vi "Grab.vi"() -> ()   [LabVIEW 2017]
doc: "The Grab VI acquires images continuously and displays the images in an image control using high-level acquisition VIs. A grab is appropriate for high-speed applications in which you need to process only one image at a time."
uses:
  <vilib>/vision/driver/NI_Vision_Acquisition_Software.lvlib
panel:
  in  "UI电源线正面标签1参数 2":T2={"Rectangle"={"Left"=1066, "Top"=596, "Right"=370, "Bottom"=2690, "Rotation"=45.0}, "Angle (degrees) (Geometry 1)"=90.0, "中心位置"={"Cent X"=273.0, "Cent Y"=255.0, "半径"=300.0}, "long"=150.0, "abgek"=-90.0, "Color"=16711680, "left threshold"=0.0, "Rectangle right"={"Left"=1066, "Top"=1096, "Right"=570, "Bottom"=2690, "Rotation"=45.0}, "long right"=150.0, "abgek right"=90.0, "Color 2"=16711680, "right threshold"=0.0, "left"=0.0, "right"=0.0} {"Rectangle right"."Rotation" format="%.2f"; "Rectangle right"."Left" scale=0.0..1024.0; "Rectangle right"."Right" scale=0.0..1024.0; "Rectangle"."Rotation" format="%.2f"; "Rectangle"."Left" scale=0.0..1024.0; "Rectangle"."Right" scale=0.0..1024.0}
  out "输出簇":T3={"Clamp Points (Max Clamp 1)"={"Pixels "={"Start"={"X"=804.5, "Y"=852.5074462890625}, "End"={"X"=804.5, "Y"=932.54296875}}, "Real World"={"Start"={"X"=804.5, "Y"=852.5074462890625}, "End"={"X"=804.5, "Y"=932.54296875}}}, "Clamp Points (Max Clamp 2)"={"Pixels "={"Start"={"X"=1018.1555786132812, "Y"=879.031982421875}, "End"={"X"=1027.8096923828125, "Y"=907.3988647460938}}, "Real World"={"Start"={"X"=1018.1555786132812, "Y"=879.031982421875}, "End"={"X"=1027.8096923828125, "Y"=907.3988647460938}}}}
  in  "布尔":bool
  in  "等待时间（毫秒）":u32
  out "error out":errorcluster={"status"=TRUE, "code"=-1074396120, "source"="IMAQ WriteJPEGFile\n  "}
  in  "error in (no error)":errorcluster
  out "连接的字符串":string="\\20181121\\CCD2\\Image\\11_24_49.jpeg"
  in  "Camera Name":refnum<k21> caption="IMAQdx Session"
  out "Buffer Number":u32
  out "Image":T4(plugin-control)
  out "Frame Rate":dbl(knob) scale=0.0..100.0
  in  "Stop":bool
  # "Overview: Demonstrates how to acquire images continuously using a Grab acquisition.\nRequirements: Vision Acquisition Software\nInstructions: \n1. Select the Camera Name.\n2. Run the VI"
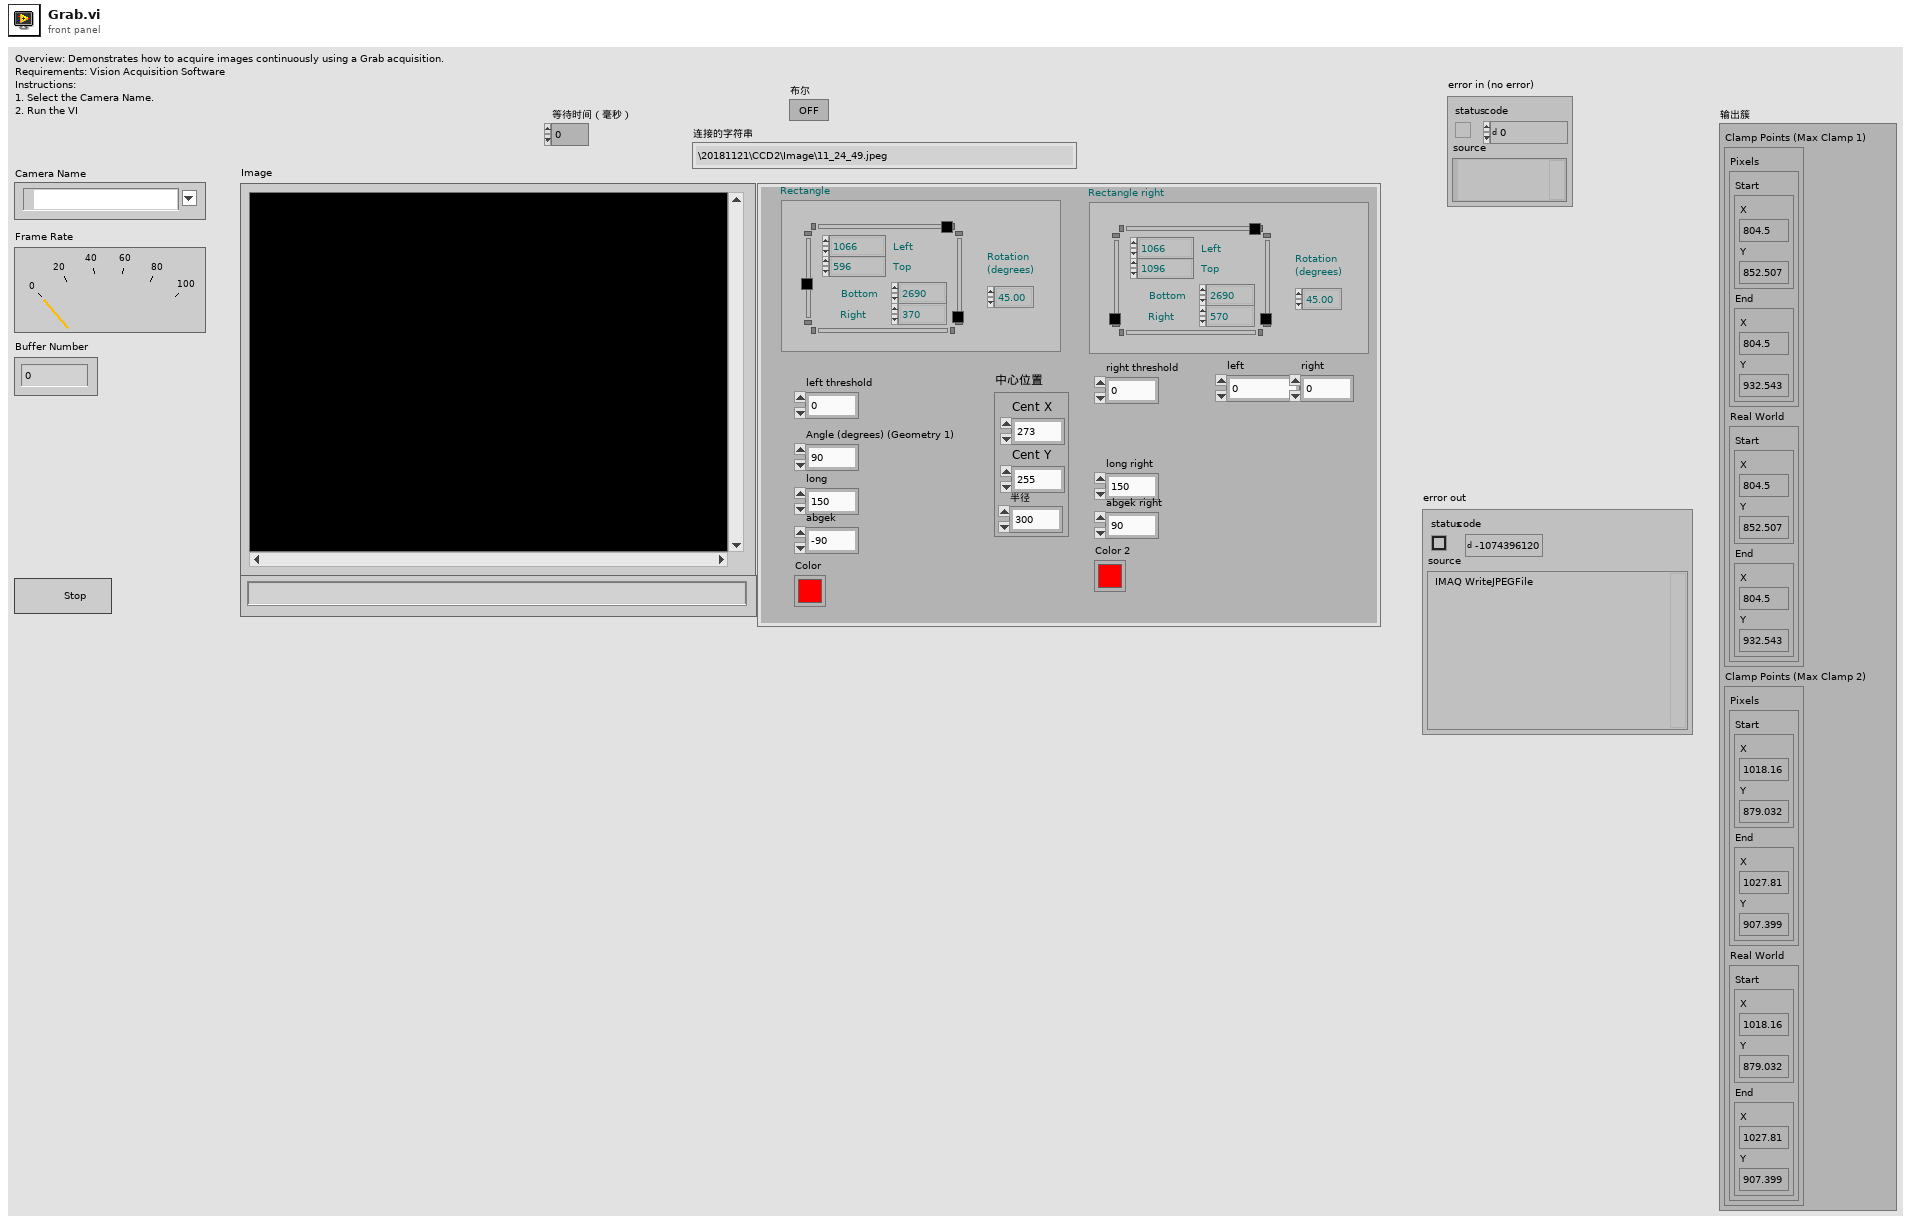
[diagram p1: front panel]
types:
  T1 = typedef "IMAQ Rectangle" = cluster{"Left":i32, "Top":i32, "Right":i32, "Bottom":i32, "Rotation":dbl}
  T2 = cluster{"Rectangle":T1, "Angle (degrees) (Geometry 1)":sgl, "中心位置":cluster{"Cent X":dbl, "Cent Y":dbl, "半径":dbl}, "long":sgl, "abgek":dbl, "Color":u32, "left threshold":dbl, "Rectangle right":T1, "long right":sgl, "abgek right":dbl, "Color 2":u32, "right threshold":dbl, "left":dbl, "right":dbl}
  T3 = cluster{"Clamp Points (Max Clamp 1)":cluster{"Pixels ":cluster{"Start":cluster{"X":dbl, "Y":dbl}, "End":cluster{"X":dbl, "Y":dbl}}, "Real World":cluster{"Start":cluster{"X":dbl, "Y":dbl}, "End":cluster{"X":dbl, "Y":dbl}}}, "Clamp Points (Max Clamp 2)":cluster{"Pixels ":cluster{"Start":cluster{"X":dbl, "Y":dbl}, "End":cluster{"X":dbl, "Y":dbl}}, "Real World":cluster{"Start":cluster{"X":dbl, "Y":dbl}, "End":cluster{"X":dbl, "Y":dbl}}}}
  T4 = typedef "IMAQ Image.ctl" = refnum<image>
  T5 = typedef "IMAQdx.ctl" = refnum<k21>
  T6 = cluster{"Pixels ":cluster{"Start":cluster{"X":dbl, "Y":dbl}, "End":cluster{"X":dbl, "Y":dbl}}, "Real World":cluster{"Start":cluster{"X":dbl, "Y":dbl}, "End":cluster{"X":dbl, "Y":dbl}}}
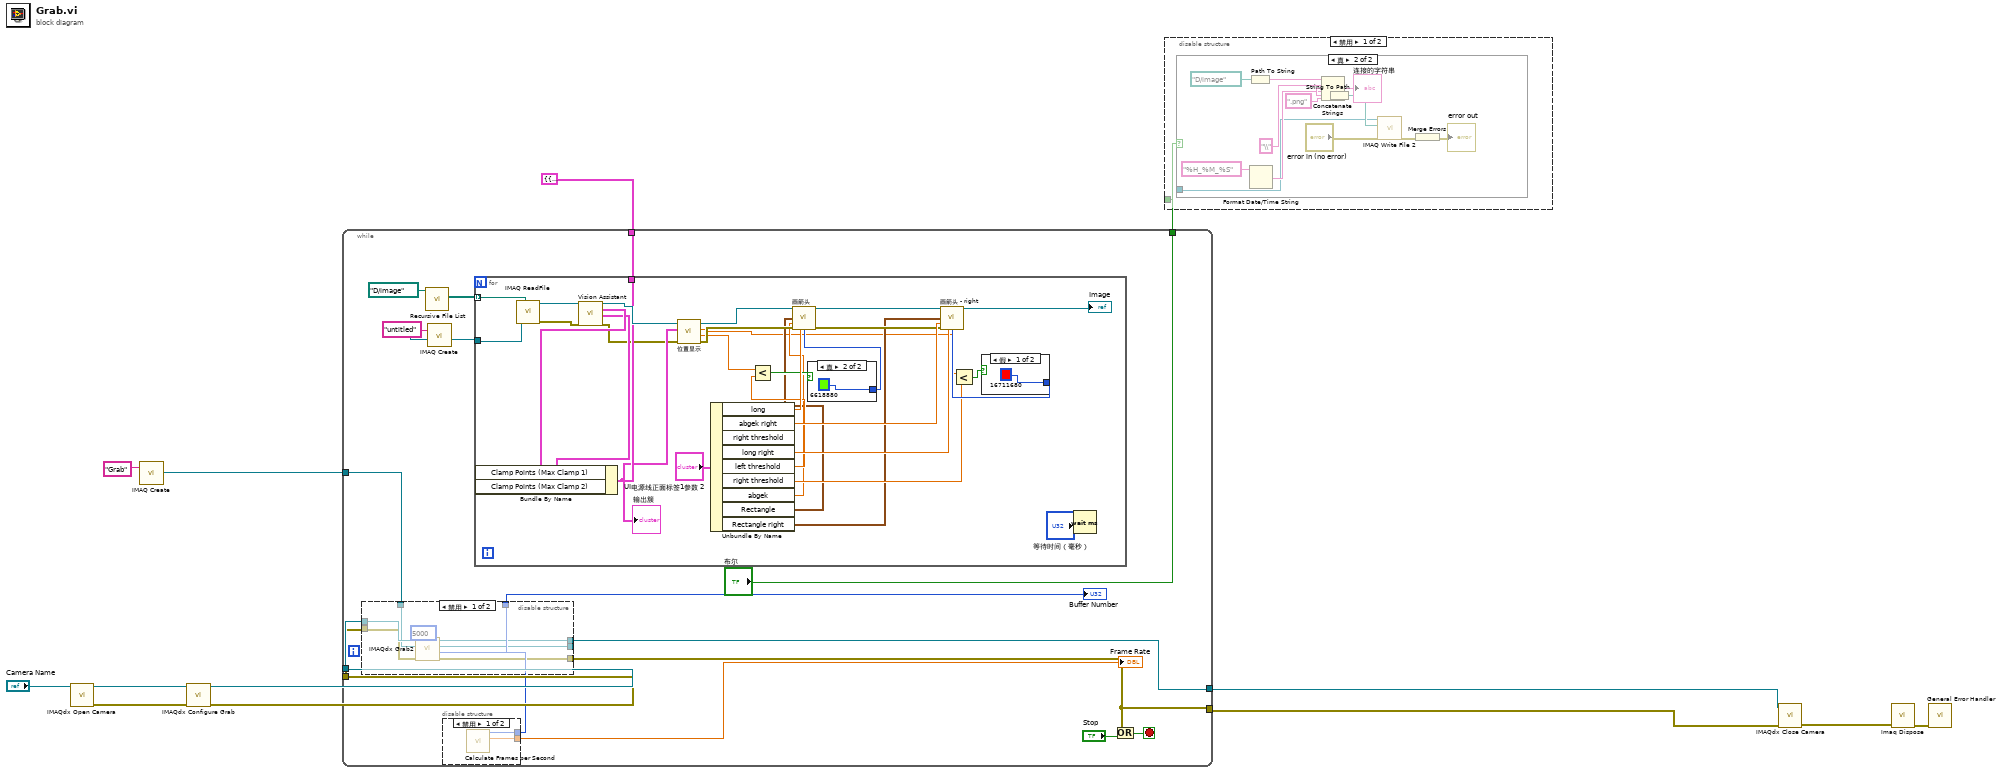
[diagram p0: block diagram]
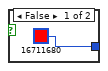
[diagram p4: hidden frame]
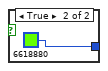
[diagram p5: hidden frame]
diagram:
  n1 = call <vilib>:"IMAQdx Open Camera.vi"("Session In"="Camera Name") -> ("error out"=w9:errorcluster, "Session Out"=w8:T5)  [unwired: 2 in, 7 out]
  n2 = call "IMAQ Create"("Image Name"="Grab") -> ("New Image"=w13:T4)  [unwired: 3 in, 2 out]
  n3 = call <vilib>:"IMAQdx Configure Grab.vi"("error in"=w9, "Session In"=w8) -> ("error out"=w11:errorcluster, "Session Out"=w12:T5)  [unwired: 8 out]
  n4 = while {
    tunnel: [w20] -> w3
    tunnel: w11 -> [w25]
    tunnel: w12 -> [w26]
    tunnel: [w21] -> w10
    tunnel: w13 -> [w24]
    tunnel: T3 {"Clamp Points (Max Clamp 1)"={"Pixels "={"Start"={"X"=0.0, "Y"=0.0}, "End"={"X"=0.0, "Y"=0.0}}, "Real World"={"Start"={"X"=0.0, "Y"=0.0}, "End"={"X"=0.0, "Y"=0.0}}}, "Clamp Points (Max Clamp 2)"={"Pixels "={"Start"={"X"=0.0, "Y"=0.0}, "End"={"X"=0.0, "Y"=0.0}}, "Real World"={"Start"={"X"=0.0, "Y"=0.0}, "End"={"X"=0.0, "Y"=0.0}}}} ("簇") -> [w15]
    tunnel: ["布尔"] -> w1
    stop <- w28 stop-if-true
    n5 = disable-structure shown="禁用" {
      disable-tunnel: w26 -> [w71 _]
      disable-tunnel: w25 -> [w70 _]
      disable-tunnel: w24 -> [w69 _]
      disable-tunnel: [w68 _] -> w22
      disable-tunnel: [w67 _] -> w21
      disable-tunnel: [w66 _] -> w20
      disable-tunnel: [w64 _] -> _
      frame Disabled {
        n6 = call <vilib>:"IMAQdx Grab2.vi"("Timeout (ms)"=5000, "error in"=w70, "Image In"=w69, "Session In"=w71) -> ("error out"=w67:errorcluster, "Buffer Number Out"=w68:u32, "Image Out"=w64:T4, "Session Out"=w66:T5)  [unwired: 4 in]
      }
      frame Enabled {
      }
    }
    "Buffer Number" <- w22
    n7 = call <vilib>:"Recursive File List.vi"("Folder Path"=path "D:/image") -> ("All Files in Dir"=w18:path[])  [unwired: 6 in, 4 out]
    n8 = call "IMAQ Create"("Image Name"="untitled") -> ("New Image"=w16:T4)  [unwired: 4 in, 1 out]
    n9 = disable-structure shown="禁用" {
      disable-tunnel: [w73 _] -> w23
      disable-tunnel: w22 -> [w72 _]
      frame Disabled {
        n10 = call <vilib>:"Calculate Frames per Second.vi"("Buffer Number"=w72) -> ("Processed Frames/s"=w73:dbl)  [unwired: 8 in, 2 out]
      }
      frame Enabled {
      }
    }
    "Frame Rate" <- w23
    n11 = for {
      tunnel: w18 -> [w59] mode=indexing
      tunnel: w16 -> [w58]
      tunnel: w15 -> [w53]
      n12 = call "IMAQ ReadFile"("File Path"=w59, "Image"=w58) -> ("error out"=w56:errorcluster, "Image Out"=w57:T4)  [unwired: 5 in, 3 out]
      n13 = call "Vision Assistant"("Image In"=w57, "error in"=w56) -> ("Image Out"=w54:T4, "Clamp Points (Max Clamp 1)"=w52:T6, "Clamp Points (Max Clamp 2)"=w51:T6, "error out"=w41:errorcluster)  [unwired: 20 in, 2 out]
      n14 = Bundle By Name(cluster=w53, "Clamp Points (Max Clamp 1)"=w52, "Clamp Points (Max Clamp 2)"=w51) -> (w50:T3)
      "输出簇" <- w50
      n15 = call "位置显示.vi"("error in (no error)"=w41, "簇"=w50, "Image in"=w54) -> ("error out"=w40:errorcluster, "下"=w29:dbl, "上"=w30:dbl, "Image out"=w45:T4)  [unwired: 5 in]
      n16 = Unbundle By Name("UI电源线正面标签1参数 2") -> ("long"=w38:sgl, "abgek right"=w42:dbl, "long right"=w37:sgl, "left threshold"=w35:dbl, "right threshold"=w34:dbl, "abgek"=w33:dbl, "Rectangle"=w32:T1, "Rectangle right"=w31:T1)  [unwired: 1 out]
      n17 = Less?(x=w29, y=w35) -> (x < y?=w36:bool)
      n18 = case shown="真" w36 {
        tunnel: [u32 16711680 ("Color") u32 6618880 ("Color")] -> w47
        frame False {
        }
        frame True {
        }
      }
      n19 = call "画箭头.vi"("Image 2"=w45, "Rectangle"=w32, "abgek"=w33, "error in (no error)"=w40, "long"=w38, "Color 2"=w47) -> ("Image"=w44:T4, "error out"=w39:errorcluster)  [unwired: 8 in]
      n20 = Less?(x=w30, y=w34) -> (x < y?=w49:bool)
      n21 = case shown="假" w49 {
        tunnel: [u32 16711680 ("Color") u32 6618880 ("Color")] -> w48
        frame False {
        }
        frame True {
        }
      }
      n22 = call "画箭头 - right.vi"("Image 2"=w44, "Rectangle"=w31, "abgek"=w42, "error in (no error)"=w39, "long"=w37, "Color 2"=w48) -> ("Image"=→"Image":T4)  [unwired: 8 in, 1 out]
      n23 = Wait (ms)(milliseconds to wait="等待时间（毫秒）") -> ()  [unwired: 1 out]
    }
    n24 = Or(x=w21, y="Stop") -> (x .or. y?=w28:bool)
  }
  n25 = disable-structure shown="禁用" {
    disable-tunnel: w1 -> [w74 _]
    frame Disabled {
      n26 = case shown="真" w74 {
        tunnel: _ -> [_ w75]
        frame False {
        }
        frame True {
          n27 = Path To String(path=path "D:/image" ("基路径")) -> (string=w78:string)
          n28 = Format Date/Time String(time format string (%c)="%H_%M_%S" ("时间格式字符串(%c)")) -> (date/time string=w76:string)  [unwired: 2 in]
          n29 = Concatenate Strings(w78, "\\" ("字符串"), w76, ".png" ("字符串")) -> (w82:string)
          "连接的字符串" <- w82
          n30 = String To Path(string=w82) -> (path=w79:path)
          n31 = call-poly "IMAQ Write File 2"("error in (no error)"="error in (no error)", "File Path"=w79, "Image"=w75) -> ("error out"=w85:errorcluster)  [unwired: 7 in, 1 out]
          n32 = Merge Errors(w85) -> (→"error out":errorcluster)
        }
      }
    }
    frame Enabled {
    }
  }
  n33 = call <vilib>:"IMAQdx Close Camera.vi"("error in"=w10, "Session In"=w3) -> ("error out"=w6:errorcluster)  [unwired: 9 out]
  n34 = call "Imaq Dispose"("error in (no error)"=w6) -> ("error out"=w5:errorcluster)  [unwired: 5 in]
  n35 = call <vilib>:"General Error Handler.vi"("error in (no error)"=w5) -> ()  [unwired: 2 in, 13 out]
